vi "Engine - Generic - Direct Injector Host.vi"() -> ()   [LabVIEW 2015, in "ECS-Host.lvlib"]
uses:
  ECS-Host.lvlib
  <vilib>/addons/Software Calibration Management/XControls/TBL2D.xctl
panel:
  in  "FuelDensity":sgl caption="[kg/m3]"
  in  "MinInjDur":sgl caption="[]"
  in  "MaxInjDur":sgl caption="[ms]"
  out "_Pulse Index 2":string[](array[string]) caption="[]"
  in  "DIWindowEnd":sgl caption="[]"
  in  "DIWindowStart":sgl caption="[]"
  out "_Pulse Gen Labels Row 2":string[](array[string]) caption="[]"
  out "Inj1Duration":sgl[](array[numeric]) caption="[msec]" format="%#.3g"
  out "Inj2Duration":sgl[](array[numeric]) caption="[msec]" format="%#.3g"
  out "Inj3Duration":sgl[](array[numeric]) caption="[msec]" format="%#.3g"
  out "Inj4Duration":sgl[](array[numeric]) caption="[msec]" format="%#.3g"
  out "Inj5Duration":sgl[](array[numeric]) caption="[msec]" format="%#.3g"
  out "Inj6Duration":sgl[](array[numeric]) caption="[msec]" format="%#_3g"
  out "Inj7Duration":sgl[](array[numeric]) caption="[msec]" format="%#.3g"
  out "Inj8Duration":sgl[](array[numeric]) caption="[msec]" format="%#.3g"
  in  "Pilot1Dur_ManE":bool caption="Enable Inj"
  in  "Post2Dur_Man":sgl caption="[]"
  in  "Post1Dur_Man":sgl caption="[]"
  in  "MainDur_Man":sgl caption="[]"
  in  "Pilot2Dur_Man":sgl caption="[]"
  in  "Pilot1Dur_Man":sgl caption="[msec]"
  in  "Post2Dur_ManE":bool caption="Enable Inj"
  in  "Post1Dur_ManE":bool caption="Enable Inj"
  in  "MainDur_ManE":bool caption="Enable Inj"
  in  "Pilot2Dur_ManE":bool caption="Enable Inj"
  out "Inj1Timing":sgl[](array[numeric]) caption="[DBTDC]" format="%#.3g"
  out "Inj2Timing":sgl[](array[numeric]) caption="[DBTDC]" format="%#.3g"
  out "Inj3Timing":sgl[](array[numeric]) caption="[DBTDC]" format="%#.3g"
  out "Inj4Timing":sgl[](array[numeric]) caption="[DBTDC]" format="%#.3g"
  out "Inj5Timing":sgl[](array[numeric]) caption="[DBTDC]" format="%#.3g"
  out "Inj6Timing":sgl[](array[numeric]) caption="[DBTDC]" format="%#.3g"
  out "Inj7Timing":sgl[](array[numeric]) caption="[DBTDC]" format="%#.3g"
  out "Inj8Timing":sgl[](array[numeric]) caption="[DBTDC]" format="%#.3g"
  out "_Pulse Index":string[](array[string]) caption="[]"
  out "_Pulse Gen Labels Row 1":string[](array[string]) caption="[]"
  in  "_DI_Inj_Enable":bool[](array[boolean])
  in  "InjPulseSwitch":u8
  in  "InjCalibration_Tbl":cluster{"X":sgl[], "Y":sgl[], "Z":sgl[][]}(xcontrol) caption="[]"
  # "Fuel Pressure"
  # "Fuel Quantity"
  # "DI Driver 1-4"
  # "DI Driver 1-4"
  # "Manual Injection Durations"
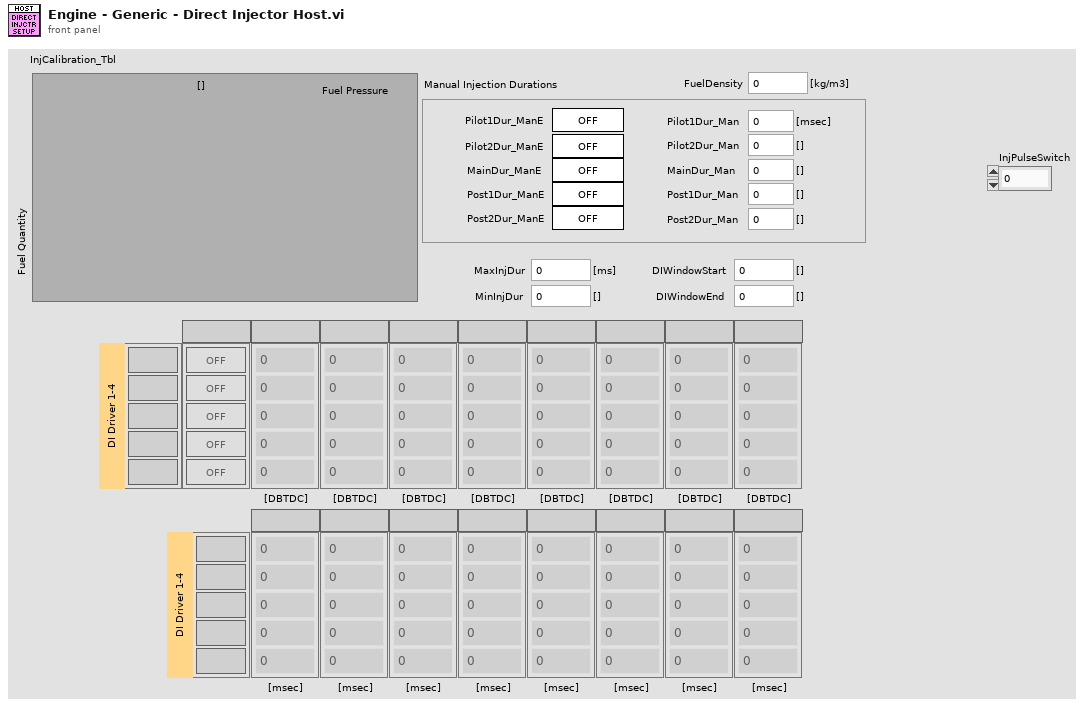
[diagram p1: front panel]
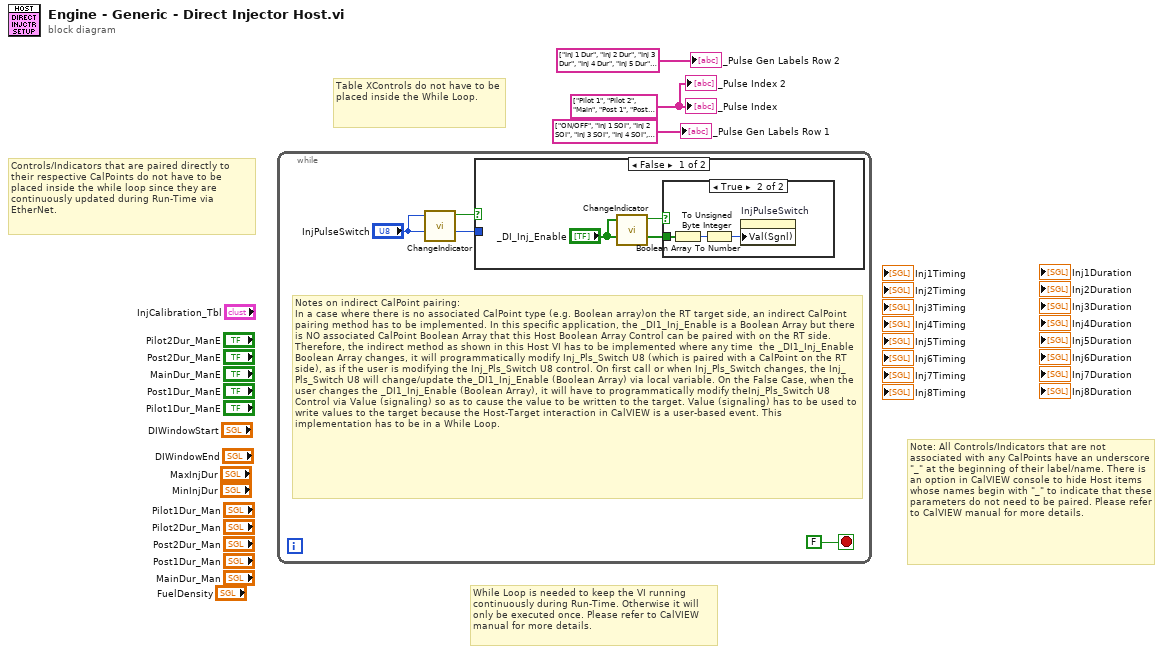
[diagram p0: block diagram]
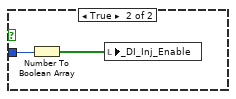
[diagram p3: hidden frame]
diagram:
  w3 = string[] ["Pilot 1", "Pilot 2", "Main", "Post 1", "Post 2"] ("DIFuelDurationArray 2")
  # "Controls/Indicators that are paired directly to their respective CalPoints do not have to be placed inside the while loop since they are continuously updated during Run-Time via EtherNet."
  # "Table XControls do not have to be placed inside the While Loop."
  # "While Loop is needed to keep the VI running\ncontinuously during Run-Time. Otherwise it will only be executed once. Please refer to CalVIEW manual for more details."
  # "Note: All Controls/Indicators that are not associated with any CalPoints have an underscore \"_\" at the beginning of their label/name. There is an option in CalVIEW console to hide Host items whose names begin with \"_\" to indicate that these parameters do not need to be paired. Please refer to CalVIEW manual for more details."
  n1 = while {
    stop <- FALSE stop-if-true
    # "Notes on indirect CalPoint pairing:\nIn a case where there is no associated CalPoint type (e.g. Boolean array)on the RT target side, an indirect CalPoint pairing method has to be implemented. In this specific application, the _DI1_Inj_Enable is a Boolean Array but there is NO associated CalPoint Boolean Array that this Host Boolean Array Control can be paired with on the RT side. Therefore, the indirect method as shown in this Host VI has to be implemented where any time  the _DI1_Inj_Enable Boolean Array changes, it will programmatically modify Inj_Pls_Switch U8 (which is paired with a CalPoint on the RT side), as if the user is modifying the Inj_Pls_Switch U8 control. On first call or when Inj_Pls_Switch changes, the Inj_Pls_Switch U8 will change/update the_DI1_Inj_Enable (Boolean Array) via local variable. On the False Case, when the user changes the _DI1_Inj_Enable (Boolean Array), it will have to programmatically modify theInj_Pls_Switch U8 Control via Value (signaling) so as to cause the value to be written to the target. Value (signaling) has to be used to write values to the target because the Host-Target interaction in CalVIEW is a user-based event. This implementation has to be in a While Loop."
    n2 = call "ChangeIndicator.vi"("Input"="InjPulseSwitch") -> ("Change"=w4:bool)  [unwired: 9 in]
    n3 = case shown="False" w4 {
      tunnel: "InjPulseSwitch" -> [_ w13]
      frame False {
        n4 = call "ChangeIndicator.vi"("Input"="_DI_Inj_Enable") -> ("Change"=w8:bool)  [unwired: 9 in]
        n5 = case shown="True" w8 {
          tunnel: "_DI_Inj_Enable" -> [_ w11]
          frame False {
          }
          frame True {
            n6 = Boolean Array To Number(Boolean array=w11) -> (number=w10:u32)
            n7 = To Unsigned Byte Integer(number=w10) -> (unsigned 8bit integer=w9:u8)
            n8 = property on="InjPulseSwitch" class="DigNum (strict)"("Val(Sgnl)"=w9) -> ()  [unwired: 2 in, 2 out]
          }
        }
      }
      frame True {
        n9 = Number To Boolean Array(number=w13) -> (Boolean array=w12:bool[])
        n10 = local write "_DI_Inj_Enable"(w12) -> ()
      }
    }
  }
  "_Pulse Index" <- w3
  "_Pulse Gen Labels Row 1" <- string[] ["ON/OFF", "Inj 1 SOI", "Inj 2 SOI", "Inj 3 SOI", "Inj 4 SOI", "Inj 5 SOI", "Inj 6 SOI", "Inj 7 SOI", "Inj 8 SOI"] ("_Pulse Gen Labels 2")
  "_Pulse Gen Labels Row 2" <- string[] ["Inj 1 Dur", "Inj 2 Dur", "Inj 3 Dur", "Inj 4 Dur", "Inj 5 Dur", "Inj 6 Dur", "Inj 7 Dur", "Inj 8 Dur"] ("_Pulse Gen Labels 2")
  "_Pulse Index 2" <- w3
